vi "PCO_GetCameraRamSegmentSize.vi"(8 "error in (no error)":errorcluster {"code" format="%x"}, 11 "ph":u64) -> (0 "error out":errorcluster {"code" format="%x"}, 1 "dwRamSegSize":u32[](array[numeric]), 2 "ErrorMessage":i32 format="%x", 3 "ph out":u64)   [LabVIEW 2019, in "SDK.lvlib" / "StorageControl.lvlib"]
doc: "<b>Description:</b>\nThis function returns a list of memory segment sizes in CamRAM pages.\n\n<b>Supported camera type:</b>\npco.dimax, pco.1200, pco.1600, pco.2000, pco.4000\n\n<b>Descriptor dependency:</b>\ndwGeneralCapsDESC1: NO_RECORDER"
uses:
  StorageControl.lvlib
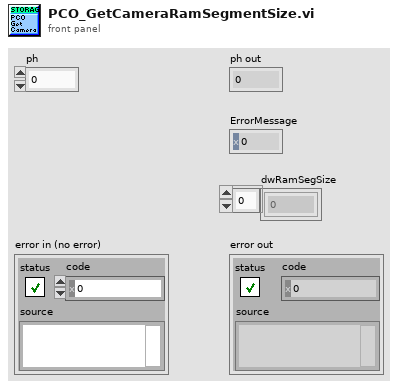
[diagram p1: front panel]
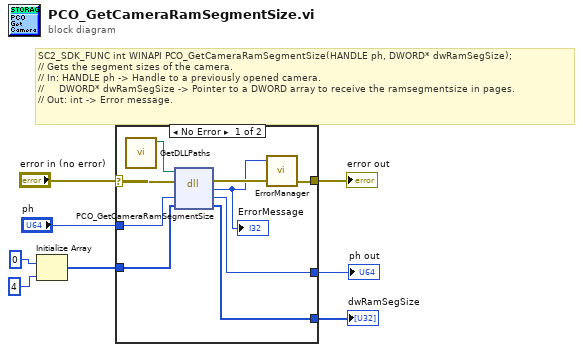
[diagram p0: block diagram]
diagram:
  # "SC2_SDK_FUNC int WINAPI PCO_GetCameraRamSegmentSize(HANDLE ph, DWORD* dwRamSegSize);\n// Gets the segment sizes of the camera.\n// In: HANDLE ph -> Handle to a previously opened camera.\n//     DWORD* dwRamSegSize -> Pointer to a DWORD array to receive the ramsegmentsize in pages.\n// Out: int -> Error message."
  n1 = Initialize Array(u32 0 ("dwRamSegSize"), 4 ("dimension size")) -> (w2:u32[])
  n2 = case shown="No Error" "error in (no error)" {
    selector: "error in (no error)" -> [w13 w20]
    tunnel: "ph" -> [w17 w19]
    tunnel: [w16 w19] -> w7
    tunnel: [w11 w20] -> w6
    tunnel: [w15 w18] -> w5
    tunnel: w2 -> [w14 w18]
    frame No Error {
      n3 = call "GetDLLPaths.vi"() -> ("SC2_Cam_Path"=w9:path)  [unwired: 8 in, 3 out]
      n4 = dll-call lib="?" fn="PCO_GetCameraRamSegmentSize"(path in=w9, error in=w13, "ph"=w17, "dwRamSegSize"=w14) -> (error out=w12:errorcluster, "return type"=w10:i32, "ph"=w16:u64, "dwRamSegSize"=w15:u32[])  [unwired: 1 in, 1 out]
      "ErrorMessage" <- w10
      n5 = call "ErrorManager.vi"("error in (no error)"=w12, "error code"=w10) -> ("error out"=w11:errorcluster)  [unwired: 2 in, 1 out]
    }
    frame Error {
    }
  }
  "ph out" <- w7
  "error out" <- w6
  "dwRamSegSize" <- w5
